vi "RehomeArm.vi"(11 "Buttons":bool[](array[boolean])) -> ()   [LabVIEW 2015]
uses:
  <vilib>/Rock Robotics/WPI/CAN/TalonSRX/WPI_CANTalonSRX_APIControlMode.ctl
  <vilib>/Rock Robotics/WPI/CAN/TalonSRX/WPI_CANTalonSRX_APIFeedbackSelect.ctl
panel:
  in  "Arm PID Gains":T1={"proportional gain (Kc)"=2.0, "integral time (Ti, min)"=0.0, "derivative time (Td, min)"=6.0}
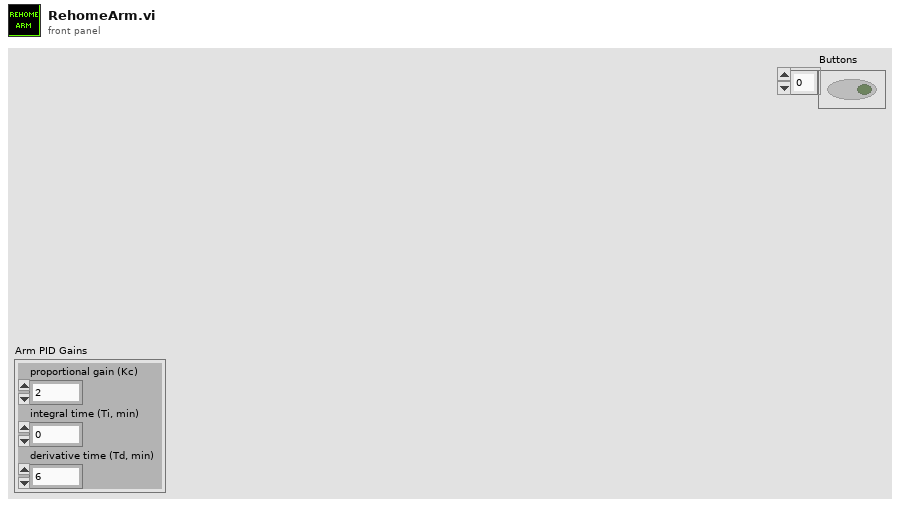
[diagram p1: front panel]
types:
  T1 = cluster{"proportional gain (Kc)":dbl, "integral time (Ti, min)":dbl, "derivative time (Td, min)":dbl}
  T2 = typedef "WPI_CANTalonSRX_APIControlMode.ctl" = enum8{"Percent VBus", "Speed", "Position", "Slave", "Unchanged / Invalid", "Voltage Compensation", "Current", "Motion Profile"}
  T3 = typedef "WPI_CANTalonSRX_APIFeedbackSelect.ctl" = enum16{"Digital Quadrature Encoder", "Analog Potentiometer", "Analog Encoder", "Count on Quad-A (Rising-Edge)", "Count on Quad-A (Falling-Edge)", "CTR Magnetic Enc (Absolute)", "CTR Magnetic Enc (Relative)", "Pulse Width"}
  T4 = typedef "WPI_MotorControlDeviceRef.ctl" = cluster{"DeviceStatus":errorcluster, "Type":T5, "PWM":cluster{"PWM Channel":T6, "DeadBand":T7}, "CAN":cluster{"Device Number":u8, "Control Mode":T8, "Semaphore":T9, "Max Vout":dbl, "TalonSRX Control Mode":T2}, "Invert":bool}
  T5 = typedef "WPI_MotorControlType.ctl" = enum16{"PWM", "CAN", "CANTalonSRX"}
  T6 = typedef "FPGA_DIOPWMChannel.ctl" = enum8{"PWM 0", "PWM 1", "PWM 2", "PWM 3", "PWM 4", "PWM 5", "PWM 6", "PWM 7", "PWM 8", "PWM 9", "PWM MXP 0", "PWM MXP 1", "PWM MXP 2", "PWM MXP 3", "PWM MXP 4", "PWM MXP 5", "PWM MXP 6", "PWM MXP 7", "PWM MXP 8", "PWM MXP 9", "Invalid"}
  T7 = typedef "WPI_PWMDeadband.ctl" = cluster{"Name":string, "maxPositivePwm":i32, "minPositivePwm":i32, "centerPwm":i32, "maxNegativePwm":i32, "minNegativePwm":i32, "angularRange":u16}
  T8 = typedef "WPI_CANJaguar_ControlMode.ctl" = enum8{"Percent VBus", "Current", "Speed", "Position", "Voltage"}
  T9 = typedef "Semaphore RefNum" = refnum<k1>
  T10 = typedef "WPI_CANTalonSRX_GlobalStatus.ctl" = cluster{"Applied Throttle":dbl, "Module Enabled":bool, "CAN Error":errorcluster, "Closed Loop Error":dbl, "Forward Limit Switch Closed":bool, "Reverse Limit Switch Closed":bool, "Sensor Position":dbl, "Sensor Velocity":dbl, "Current":dbl, "Sticky Fault - Over Temp":bool, "Sticky Fault - Under Voltage":bool, "Sticky Fault - Forward Limit":bool, "Sticky Fault - Reverse Limit":bool, "Sticky Fault - Forward Soft Limit":bool, "Sticky Fault - Reverse Soft Limit":bool, "Brake is Enabled":bool, "Encoder Position":dbl, "Encoder Velocity":dbl, "Encoder Index Count":dbl, "Encoder A Pin State":bool, "Encoder B Pin State":bool, "Encoder Index Pin State":bool, "Analog In":dbl, "Analog In Velocity":dbl, "Temperature (C)":dbl, "Battery Voltage":dbl, "Control 5 Is Supported":bool, "Current Profile Slot Select":dbl, "Pos Div 8":bool, "Vel Div 4":bool, "Pulse Width Position":i32, "Pulse Width Velocity":i32, "Pulse Width Rise To Rise (us)":i32, "Pulse Width Rise To Fall (us)":i32, "Mot Prof Active Is Under Run":bool, "Mot Prof Active Has Under Run":bool, "Mot Prof Active Is Last":bool, "Mot Prof Active Velocity Only":bool, "Mot Prof Active Is Valid":bool, "Mot Prof Buffer Is Full":bool, "Mot Prof Active Profile Slot Select":i32, "Mot Prof NextID":i32, "Mot Prof Count":i32, "Mot Prof Active Velocity":dbl, "Mot Prof Active Position":dbl, "Mot Prof Output Enable":i32}
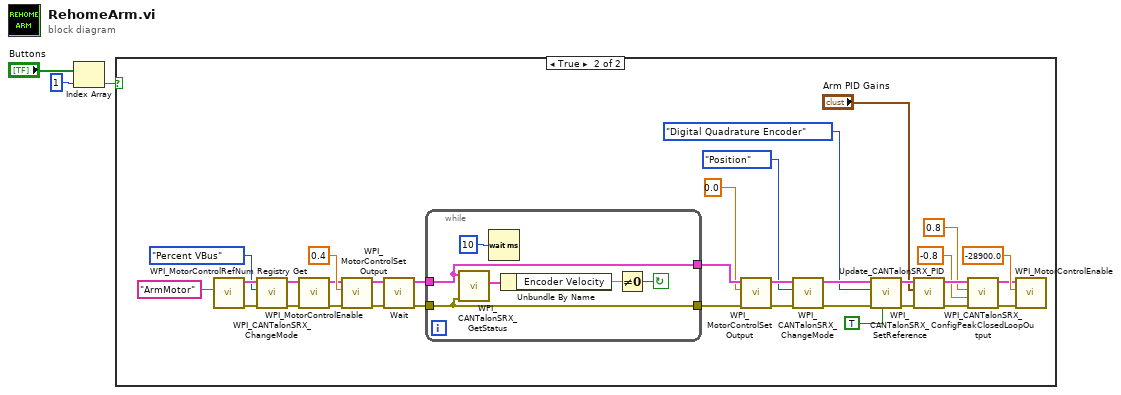
[diagram p0: block diagram]
diagram:
  n1 = Index Array(array="Buttons", index=1) -> (element=w1:bool)
  n2 = case shown="True" w1 {
    frame False {
    }
    frame True {
      n3 = call <vilib>:"WPI_MotorControlRefNum Registry Get.vi"("refnum name"="ArmMotor") -> ("error out"=w9:errorcluster, "MotorControlDevRef"=w10:T4)  [unwired: 9 in]
      n4 = call <vilib>:"WPI_CANTalonSRX_ChangeMode.vi"("error in (no error)"=w9, "Control Mode"=WPI_CANTalonSRX_APIControlMode."Percent VBus", "CAN Talon SRX Ref"=w10) -> ("error out"=w6:errorcluster, "CAN Talon SRX Ref"=w7:T4)  [unwired: 7 in]
      n5 = call <vilib>:"WPI_MotorControlEnable.vi"("error in (no error)"=w6, "CAN MotorDevRef"=w7) -> ("error out"=w4:errorcluster, "CAN MotorDevRef"=w5:T4)  [unwired: 8 in]
      n6 = call <vilib>:"WPI_MotorControlSetOutput.vi"("error in (no error)"=w4, "Output"=0.4, "MotorControlDevRef"=w5) -> ("error out"=w32:errorcluster, "MotorControlDevRef"=w33:T4)  [unwired: 6 in, 1 out]
      n7 = call "Wait.vi"("error in (no error)"=w32, "MotorControlDeviceRefIn"=w33) -> ("error out"=w30:errorcluster, "MotorControlDeviceRefOut"=w31:T4)  [unwired: 8 in]
      n8 = while {
        tunnel: w31 -> [w39]
        tunnel: [w39] -> w28
        tunnel: w30 -> [w38]
        tunnel: [w38] -> w29
        stop <- w40 continue-if-true
        n9 = call <vilib>:"WPI_CANTalonSRX_GetStatus.vi"("error in (no error)"=w38, "CAN Talon SRX Ref"=w39) -> ("Talon SRX Status"=w42:T10)  [unwired: 7 in, 2 out]
        n10 = Wait (ms)(milliseconds to wait=u32 10) -> ()  [unwired: 1 out]
        n11 = Unbundle By Name(w42) -> ("Encoder Velocity"=w41:dbl)
        n12 = Not Equal To 0?(x=w41) -> (x != 0?=w40:bool)
      }
      n13 = call <vilib>:"WPI_MotorControlSetOutput.vi"("error in (no error)"=w29, "Output"=0.0, "MotorControlDevRef"=w28) -> ("error out"=w25:errorcluster, "MotorControlDevRef"=w26:T4)  [unwired: 6 in, 1 out]
      n14 = call <vilib>:"WPI_CANTalonSRX_ChangeMode.vi"("error in (no error)"=w25, "Control Mode"=WPI_CANTalonSRX_APIControlMode."Position", "CAN Talon SRX Ref"=w26) -> ("error out"=w22:errorcluster, "CAN Talon SRX Ref"=w23:T4)  [unwired: 7 in]
      n15 = call <vilib>:"WPI_CANTalonSRX_SetReference.vi"("Reverse Closed-Loop Output"=TRUE, "error in (no error)"=w22, "Feedback Reference"=WPI_CANTalonSRX_APIFeedbackSelect."Digital Quadrature Encoder", "CAN Talon SRX Ref"=w23) -> ("error out"=w19:errorcluster, "CAN Talon SRX Ref"=w20:T4)  [unwired: 6 in]
      n16 = call "Update_CANTalonSRX_PID.vi"("error in (no error)"=w19, "PID Gains"="Arm PID Gains", "CAN Talon SRX Ref"=w20) -> ("error out"=w14:errorcluster, "CAN Talon SRX Ref Out"=w17:T4)  [unwired: 7 in]
      n17 = call <vilib>:"WPI_CANTalonSRX_ConfigPeakClosedLoopOutput.vi"("error in (no error)"=w14, "Reverse Peak Output"=-0.8, "Forward Peak Output"=0.8, "CAN Talon SRX Ref"=w17) -> ("error out"=w15:errorcluster, "CAN Talon SRX Ref"=w16:T4)  [unwired: 6 in]
      n18 = call <vilib>:"WPI_MotorControlEnable.vi"("error in (no error)"=w15, "Encoder Initial Position"=-28900.0, "CAN MotorDevRef"=w16) -> ()  [unwired: 7 in, 2 out]
    }
  }
